vi "weight_experimental7.vi"(6 "Reset":bool, 7 "Stop read":bool, 9 "<0>":bool, 10 "Tick":u32=100, 11 "PV weight":dbl caption="g" format="%#.0f") -> (0 "Vibration":bool caption="Вибрация", 2 "Q":T2 {"Q 1" format="%#.0f"; "dM 1" format="%#.0f"; "W 1" format="%#.0f"; "Q 4" format="%#.0f"; "dM 4" format="%#.0f"; "Q 3" format="%#.0f"; "dM 3" format="%#.0f"; "Q 2" format="%#.0f"; "dM 2" format="%#.0f"}, 3 "Weight filtr":dbl caption="g" format="%#.0f", 5 "This VI":refnum<vi>)   [LabVIEW 2019]
uses:
  <vilib>/Analysis/baseanly.llb/Mean (DBL).vi
  Logik/fronts.vi
  Trigers/RS.vi
  Timer Delay/Timers.lvlib
  <vilib>/Analysis/NI_AALBase.lvlib
  Userlib.lvlib
  <vilib>/ptbypt/NI_PtbyPt.lvlib
panel:
  in  "Tab Control":T1(tab)=enum."Настр Sens"
  in  "Период 2, мин":i32=5
  in  "Период 3, мин":i32=10
  in  "Период 4, мин":i32=60
  in  "Период 1, сек":i32=30
  in  "Tare":dbl caption="g" format="%#.0f"
  in  "<вес>":bool
  in  "k":dbl=1.0 caption="g" format="%#.3f"
  in  "Вес":dbl caption="g" format="%#.0f"
  in  "Период оценки скорости, с":i32=30
  in  "Период оценки вибрации, с":i32=20
  in  "Вырезать после сработки, с":i32=12
  in  "порог":dbl=1000.0
  # "(вес за период)"
  # "(расход)"
  # "Вес тары\n(полностью очистить бункер от продукта\nи запомнить PV weight или ввести вручную)."
  # "Вес тары\n(ввести фактический вес без учета тары\nили ввести k вручную)"
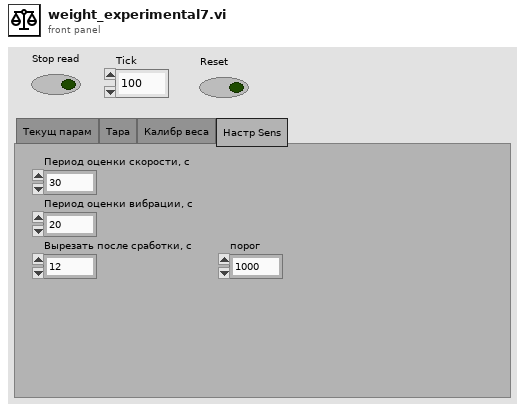
[diagram p1: front panel]
types:
  T1 = enum32{"Текущ парам", "Тара", "Калибр веса", "Настр Sens"}
  T2 = cluster{"W 1":dbl, "dM 1":dbl, "Q 1":dbl, "dM 2":dbl, "Q 2":dbl, "dM 3":dbl, "Q 3":dbl, "dM 4":dbl, "Q 4":dbl}
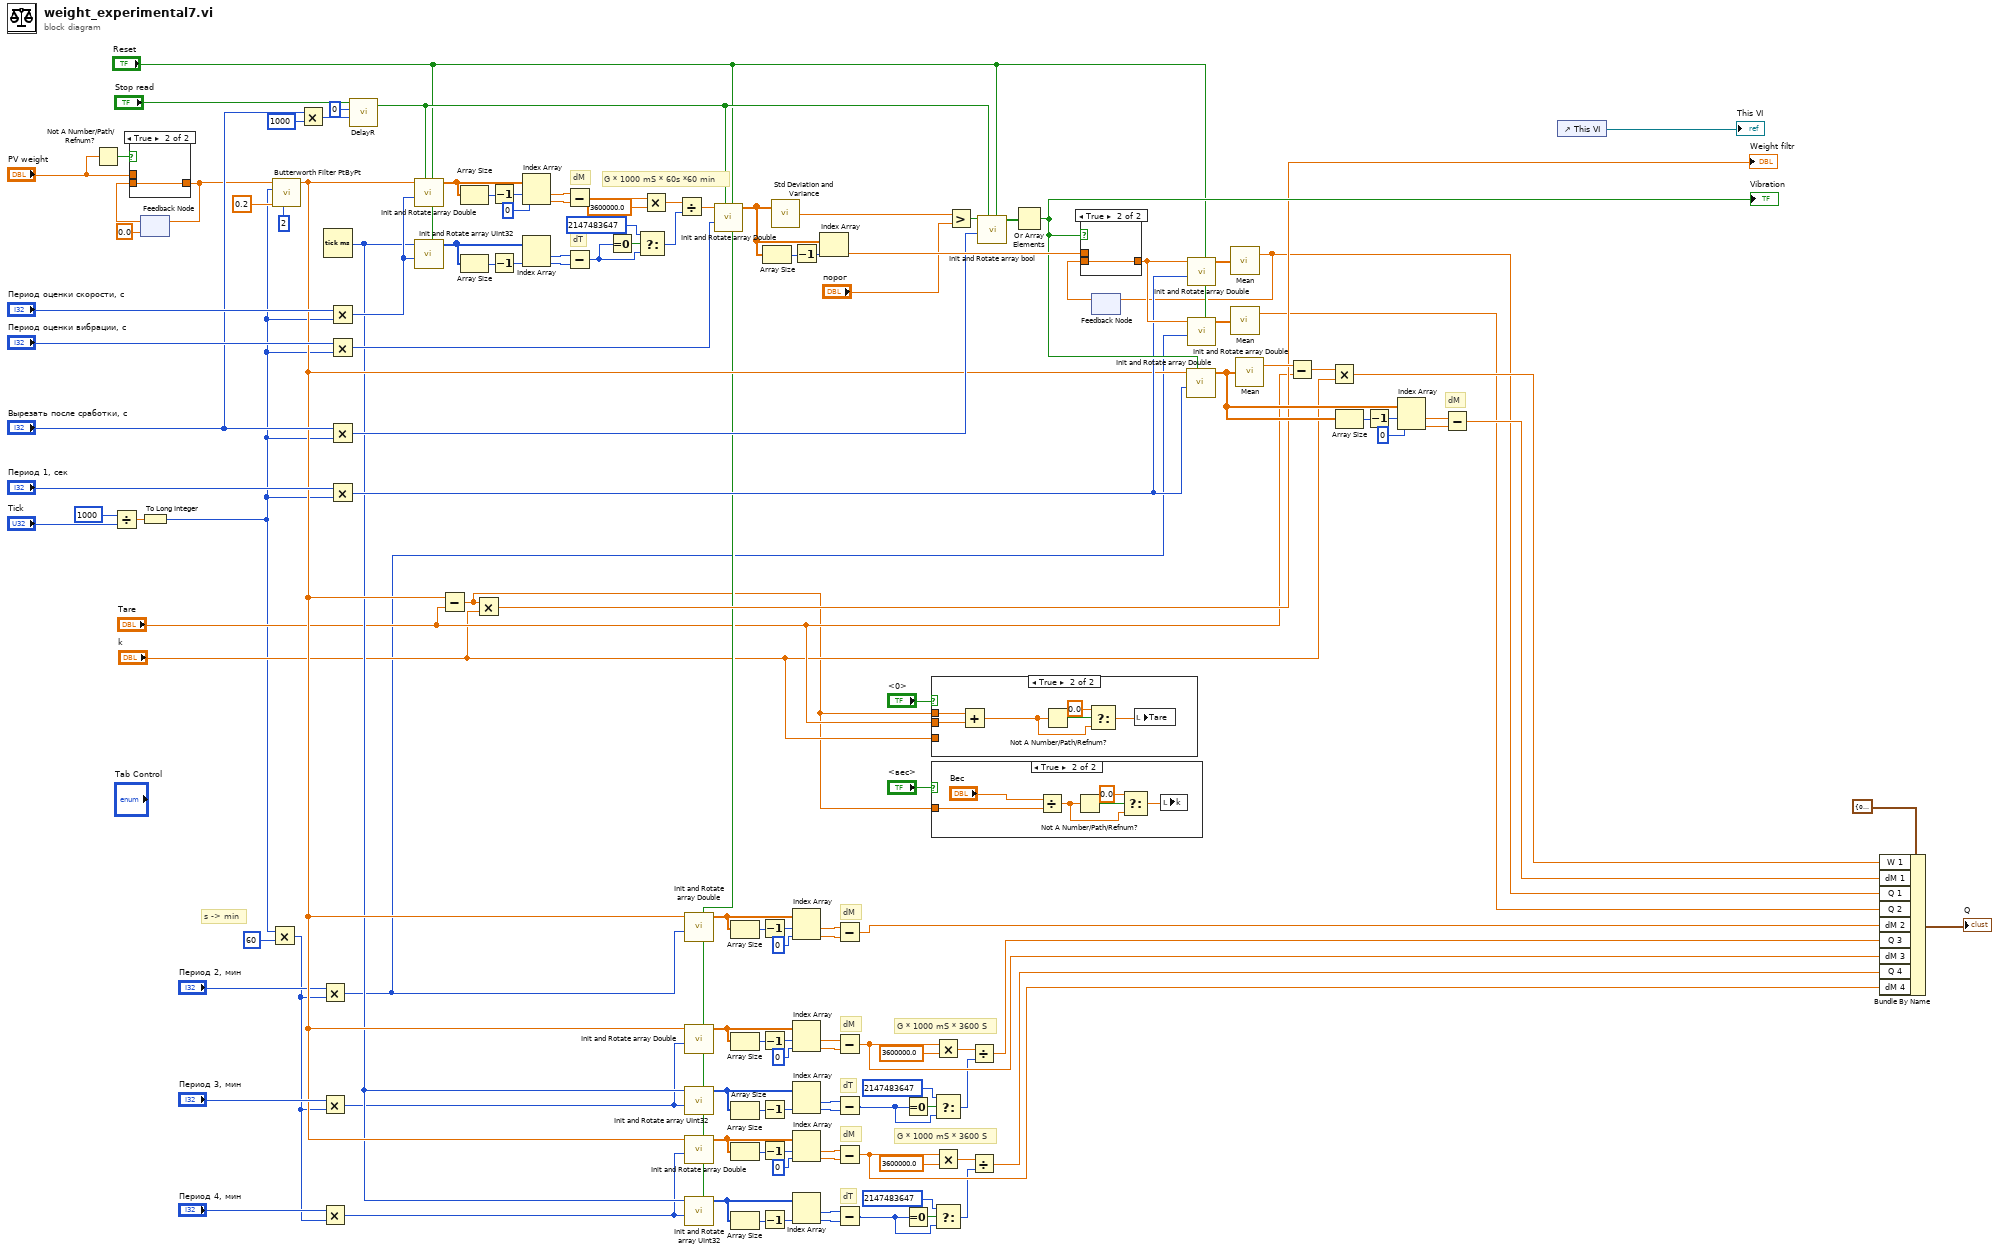
[diagram p0: block diagram]
diagram:
  # "s -> min"
  # "dT"
  # "G * 1000 mS * 3600 S"
  # "dM"
  # "dT"
  # "G * 1000 mS * 3600 S"
  # "dM"
  # "dM"
  # "dM"
  # "dT"
  # "G * 1000 mS * 60s *60 min"
  # "dM"
  n1 = Not A Number/Path/Refnum?(number/path/refnum="PV weight") -> (NaN/Path/Refnum?=w73:bool)
  n2 = Divide(x=1000 ("y"), y="Tick") -> (x/y=w89:dbl)
  n3 = feedback #1(0.0 ("PV weight")) -> (w75:dbl)
  n4 = case shown="True" w73 {
    tunnel: w75 -> [_ w135]
    tunnel: "PV weight" -> [w134 _]
    tunnel: [w134 w135] -> w76
    frame False {
    }
    frame True {
    }
  }
  n5 = feedback-in #1(w76) -> ()
  n6 = To Long Integer(number=w89) -> (32bit integer=w1:i32)
  n7 = Multiply(x=w1, y=60) -> (x*y=w8:i32)
  n8 = call <vilib>:"Butterworth Filter PtByPt.vi"("order"=2, "low cutoff freq: fl"=0.2, "sampling freq: fs"=w1, "x"=w76) -> ("Filtered x"=w36:dbl)  [unwired: 5 in, 1 out]
  n9 = Multiply(x="Вырезать после сработки, с", y=1000) -> (x*y=w105:i32)
  n10 = Multiply(x="Период 2, мин", y=w8) -> (x*y=w7:i32)
  n11 = Multiply(x="Период 3, мин", y=w8) -> (x*y=w34:i32)
  n12 = Multiply(x="Период 4, мин", y=w8) -> (x*y=w33:i32)
  n13 = Tick Count (ms)() -> (millisecond timer value=w35:u32)
  n14 = Multiply(x="Период оценки скорости, с", y=w1) -> (x*y=w84:i32)
  n15 = Multiply(x="Период оценки вибрации, с", y=w1) -> (x*y=w85:i32)
  n16 = Multiply(x="Вырезать после сработки, с", y=w1) -> (x*y=w88:i32)
  n17 = Multiply(x="Период 1, сек", y=w1) -> (x*y=w87:i32)
  n18 = call "DelayR.vi"("DelayOff"=w105, "DelayOn"=u32 0, "In"="Stop read") -> ("Out"=w100:bool)  [unwired: 1 in, 1 out]
  n19 = call "Init and Rotate array Double.vi"("Reset"="Reset", "Stop read"=w100, "Array size"=w84, "PV"=w36) -> ("Array"=w124:dbl[])  [unwired: 7 in]
  n20 = call "Init and Rotate array UInt32.vi"("Reset"="Reset", "Array size"=w84, "PV"=w35) -> ("Array"=w103:u32[])  [unwired: 8 in]
  n21 = Subtract(x=w36, y="Tare") -> (x-y=w11:dbl)
  n22 = Array Size(array=w124) -> (size(s)=w123:i32)
  n23 = Array Size(array=w103) -> (size(s)=w104:i32)
  n24 = Multiply(x=w11, y="k") -> (x*y=→"Weight filtr":dbl)
  n25 = Decrement(x=w123) -> (x-1=w120:i32)
  n26 = Decrement(x=w104) -> (x-1=w86:i32)
  n27 = Index Array(array=w124, index #1=w120, index #2=0 ("index")) -> (element #1=w122:dbl, element #2=w121:dbl)
  n28 = Index Array(array=w103, index #2=w86) -> (element #1=w102:u32, element #2=w101:u32)  [unwired: 1 in]
  n29 = Subtract(x=w122, y=w121) -> (x-y=w127:dbl)
  n30 = Subtract(x=w102, y=w101) -> (x-y=w24:u32)
  n31 = Equal To 0?(x=w24) -> (x = 0?=w25:bool)
  n32 = Select(t=u32 2147483647, s=w25, f=w24) -> (s? t:f=w23:u32)
  n33 = Multiply(x=w127, y=3600000.0) -> (x*y=w125:dbl)
  n34 = Divide(x=w125, y=w23) -> (x/y=w114:dbl)
  n35 = call "Init and Rotate array Double.vi"("Reset"="Reset", "Array size"=w7, "PV"=w36) -> ("Array"=w65:dbl[])  [unwired: 8 in]
  n36 = call "Init and Rotate array Double.vi"("Reset"="Reset", "Array size"=w34, "PV"=w36) -> ("Array"=w62:dbl[])  [unwired: 8 in]
  n37 = call "Init and Rotate array UInt32.vi"("Reset"="Reset", "Array size"=w34, "PV"=w35) -> ("Array"=w55:u32[])  [unwired: 8 in]
  n38 = call "Init and Rotate array Double.vi"("Reset"="Reset", "Array size"=w33, "PV"=w36) -> ("Array"=w41:dbl[])  [unwired: 8 in]
  n39 = call "Init and Rotate array UInt32.vi"("Reset"="Reset", "Array size"=w33, "PV"=w35) -> ("Array"=w48:u32[])  [unwired: 8 in]
  n40 = call "Init and Rotate array Double.vi"("Reset"="Reset", "Stop read"=w100, "Array size"=w85, "PV"=w114) -> ("Array"=w113:dbl[])  [unwired: 7 in]
  n41 = Array Size(array=w65) -> (size(s)=w66:i32)
  n42 = Array Size(array=w62) -> (size(s)=w61:i32)
  n43 = Array Size(array=w55) -> (size(s)=w56:i32)
  n44 = Array Size(array=w41) -> (size(s)=w42:i32)
  n45 = Array Size(array=w48) -> (size(s)=w47:i32)
  n46 = Decrement(x=w66) -> (x-1=w69:i32)
  n47 = Decrement(x=w61) -> (x-1=w58:i32)
  n48 = Decrement(x=w56) -> (x-1=w52:i32)
  n49 = Decrement(x=w42) -> (x-1=w45:i32)
  n50 = Decrement(x=w47) -> (x-1=w51:i32)
  n51 = Array Size(array=w113) -> (size(s)=w118:i32)
  n52 = call <vilib>:"Std Deviation and Variance.vi"("X"=w113) -> ("standard deviation"=w115:dbl)  [unwired: 1 in, 2 out]
  n53 = Decrement(x=w118) -> (x-1=w117:i32)
  n54 = Index Array(array=w65, index #1=w69, index #2=0 ("index")) -> (element #1=w67:dbl, element #2=w68:dbl)
  n55 = Index Array(array=w62, index #1=w58, index #2=0 ("index")) -> (element #1=w60:dbl, element #2=w59:dbl)
  n56 = Index Array(array=w55, index #2=w52) -> (element #1=w54:u32, element #2=w53:u32)  [unwired: 1 in]
  n57 = Index Array(array=w41, index #1=w45, index #2=0 ("index")) -> (element #1=w43:dbl, element #2=w44:dbl)
  n58 = Index Array(array=w48, index #2=w51) -> (element #1=w49:u32, element #2=w50:u32)  [unwired: 1 in]
  n59 = Index Array(array=w113, index=w117) -> (element=w116:dbl)
  n60 = Subtract(x=w67, y=w68) -> (x-y=w30:dbl)
  n61 = Subtract(x=w60, y=w59) -> (x-y=w27:dbl)
  n62 = Subtract(x=w54, y=w53) -> (x-y=w19:u32)
  n63 = Subtract(x=w43, y=w44) -> (x-y=w26:dbl)
  n64 = Subtract(x=w49, y=w50) -> (x-y=w15:u32)
  n65 = Equal To 0?(x=w19) -> (x = 0?=w21:bool)
  n66 = Equal To 0?(x=w15) -> (x = 0?=w17:bool)
  n67 = case shown="True" "<0>" {
    tunnel: "Tare" -> [_ w138]
    tunnel: w11 -> [_ w137]
    tunnel: "k" -> [_ _]
    frame False {
    }
    frame True {
      n68 = Add(x=w137, y=w138) -> (x+y=w136:dbl)
      n69 = Not A Number/Path/Refnum?(number/path/refnum=w136) -> (NaN/Path/Refnum?=w141:bool)
      n70 = Select(t=0.0 ("y"), s=w141, f=w136) -> (s? t:f=w139:dbl)
      n71 = local write "Tare"(w139) -> ()
    }
  }
  n72 = case shown="True" "<вес>" {
    tunnel: w11 -> [_ w142]
    frame False {
    }
    frame True {
      n73 = Divide(x="Вес", y=w142) -> (x/y=w145:dbl)
      n74 = Not A Number/Path/Refnum?(number/path/refnum=w145) -> (NaN/Path/Refnum?=w147:bool)
      n75 = Select(t=0.0 ("y"), s=w147, f=w145) -> (s? t:f=w144:dbl)
      n76 = local write "k"(w144) -> ()
    }
  }
  n77 = Multiply(x=w27, y=3600000.0) -> (x*y=w63:dbl)
  n78 = Select(t=u32 2147483647, s=w21, f=w19) -> (s? t:f=w18:u32)
  n79 = Multiply(x=w26, y=3600000.0) -> (x*y=w40:dbl)
  n80 = Select(t=u32 2147483647, s=w17, f=w15) -> (s? t:f=w14:u32)
  n81 = Greater?(x=w115, y="порог") -> (0:w112:bool)
  n82 = Divide(x=w63, y=w18) -> (x/y=w29:dbl)
  n83 = Divide(x=w40, y=w14) -> (x/y=w28:dbl)
  n84 = call "Init and Rotate array bool.vi"("Reset"="Reset", "Stop read"=w100, "Array size"=w88, "In"=w112) -> ("Array"=w111:bool[])  [unwired: 7 in]
  n85 = Or Array Elements(Boolean array=w111) -> (logical OR=w99:bool)
  "Vibration" <- w99
  n86 = feedback #2() -> (w107:dbl)  [unwired: 1 in]
  n87 = case shown="True" w99 {
    tunnel: w107 -> [_ w149]
    tunnel: w116 -> [w148 _]
    tunnel: [w148 w149] -> w108
    frame False {
    }
    frame True {
    }
  }
  n88 = call "Init and Rotate array Double.vi"("Stop read"=w99, "Array size"=w87, "PV"=w36) -> ("Array"=w94:dbl[])  [unwired: 8 in]
  n89 = call "Init and Rotate array Double.vi"("Reset"="Reset", "Array size"=w87, "PV"=w108) -> ("Array"=w110:dbl[])  [unwired: 8 in]
  n90 = call "Init and Rotate array Double.vi"("Reset"="Reset", "Array size"=w7, "PV"=w108) -> ("Array"=w109:dbl[])  [unwired: 8 in]
  n91 = call-poly <vilib>:"Mean.vi"("X"=w110) -> ("mean"=w3:dbl)  [unwired: 1 out]
  n92 = feedback-in #2(w3) -> ()
  n93 = call-poly <vilib>:"Mean.vi"("X"=w109) -> ("mean"=w2:dbl)  [unwired: 1 out]
  n94 = call-poly <vilib>:"Mean.vi"("X"=w94) -> ("mean"=w98:dbl)  [unwired: 1 out]
  n95 = Subtract(x=w98, y="Tare") -> (x-y=w130:dbl)
  n96 = Multiply(x=w130, y="k") -> (x*y=w5:dbl)
  n97 = Array Size(array=w94) -> (size(s)=w97:i32)
  n98 = Decrement(x=w97) -> (x-1=w96:i32)
  n99 = Index Array(array=w94, index #1=w96, index #2=0 ("index")) -> (element #1=w93:dbl, element #2=w92:dbl)
  n100 = Subtract(x=w93, y=w92) -> (x-y=w4:dbl)
  n101 = control-ref of="This VI"() -> (→"This VI":refnum<vi>)
  n102 = Bundle By Name(cluster=T2 {"W 1"=0.0, "dM 1"=0.0, "Q 1"=0.0, "dM 2"=0.0, "Q 2"=0.0, "dM 3"=0.0, "Q 3"=0.0, "dM 4"=0.0, "Q 4"=0.0} ("Q"), "W 1"=w5, "dM 1"=w4, "Q 1"=w3, "Q 2"=w2, "dM 2"=w30, "Q 3"=w29, "dM 3"=w27, "Q 4"=w28, "dM 4"=w26) -> (→"Q":T2)
